vi "tab_control.vi"() -> ()   [LabVIEW 2019]
panel:
  in  "Tab Control":T1(tab)
  in  "a":dbl
  in  "b":dbl
  in  "stop":bool
  out "y":dbl
  in  "x":dbl
  # "The formula calculates blah blah"
  # "Author: Vocany Pitia\nEmail: Mr.VocanyPitia@gmail.com\nDate: July 29, 2019"
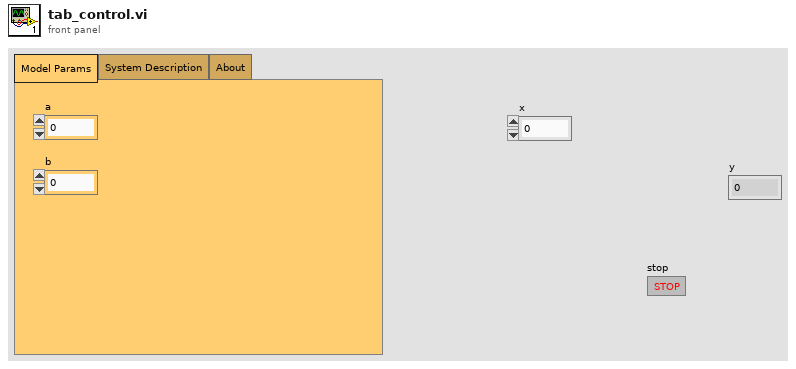
[diagram p1: front panel]
types:
  T1 = enum32{"Model Params", "System Description", "About"}
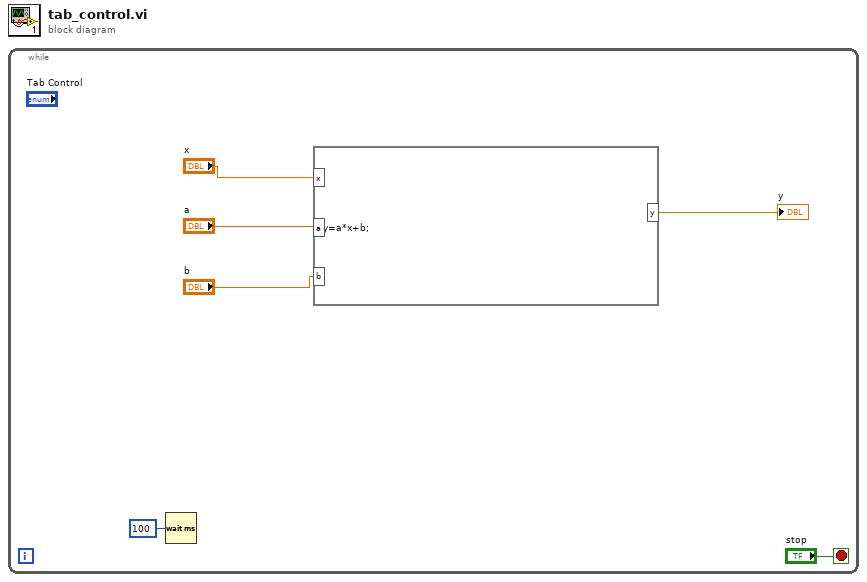
[diagram p0: block diagram]
diagram:
  n1 = while {
    stop <- "stop" stop-if-true
    n2 = Wait (ms)(milliseconds to wait=u32 100) -> ()  [unwired: 1 out]
    n3 = formula code="y=a*x+b;"("x"="x", "a"="a", "b"="b") -> ("y"=→"y":dbl)
  }
